vi "Description_parameter_type_telem_unicorn(SubVI).vi"(10 "Numeric":i32, 11 "Param":T2) -> (3 "output cluster":T1)   [LabVIEW 2017, in "LV_Unicorn.lvlib"]
uses:
  LV_Unicorn.lvlib
  Control/unicorn_DescriptParam.ctl
  Control/unicorn_Telemetry.ctl
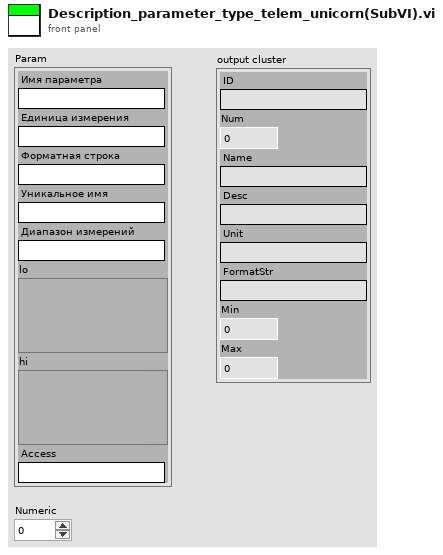
[diagram p1: front panel]
types:
  T1 = cluster{"ID":string, "Num":i32, "Name":string, "Desc":string, "Unit":string, "FormatStr":string, "Min":i32, "Max":i32}
  T2 = typedef "unicorn_DescriptParam.ctl" = cluster{"Имя параметра":string, "Единица измерения":string, "Форматная строка ":string, "Уникальное имя":string, "Диапазон измерений":string, "lo":variant, "hi":variant, "Access":string}
  T3 = typedef "LV_Unicorn.lvlib/unicorn_Telemetry.ctl" = cluster{"ID":string, "Num":i32, "Name":string, "Desc":string, "Unit":string, "FormatStr":string, "Min":i32, "Max":i32}[]
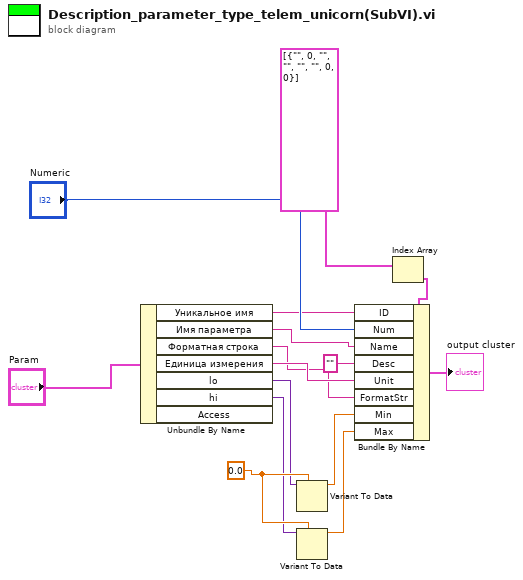
[diagram p0: block diagram]
diagram:
  w12 = sgl 0.0 ("Min")
  n1 = Unbundle By Name("Param") -> ("Уникальное имя"=w6:string, "Имя параметра"=w8:string, "Форматная строка"=w14:string, "Единица измерения"=w15:string, "lo"=w9:variant, "hi"=w11:variant)  [unwired: 1 out]
  n2 = Variant To Data(type=w12, Variant=w9) -> (data=w10:sgl)  [unwired: 1 in, 1 out]
  n3 = Variant To Data(type=w12, Variant=w11) -> (data=w13:sgl)  [unwired: 1 in, 1 out]
  n4 = Index Array(array=T3 [{"ID"="", "Num"=0, "Name"="", "Desc"="", "Unit"="", "FormatStr"="", "Min"=0, "Max"=0}] ("ParamInt 2")) -> (element=w4:T1)  [unwired: 1 in]
  n5 = Bundle By Name(cluster=w4, "ID"=w6, "Num"="Numeric", "Name"=w8, "Desc"="", "Unit"=w15, "FormatStr"=w14, "Min"=w10, "Max"=w13) -> (→"output cluster":T1)
